vi "Launch Subordinate and Add.vi"(6 "PanelIndex":i32, 7 "Identifier":string, 8 "error in (no error)":errorcluster, 9 "Panel":refnum<class "Panel.lvclass">, 10 "Nested Panel Actor":refnum<class "Panel Actor.lvclass">, 11 "Managed Actor in":refnum<class "Managed Actor.lvclass">) -> (0 "error out":errorcluster, 3 "Managed Actor out":refnum<class "Managed Actor.lvclass">)   [LabVIEW 2023, in "Engine.lvlib" / "Managed Actor.lvlib" / "Managed Actor.lvclass"]
doc: "<b>Launch Subordiate and Add</b>\nThis routine searches for an existing record of the specific subordinate being called. This prevents duplicate references to the same actor being launched.\n\nif no duplicate is found, <b>Launch Subordinate</b> is called, and the returned record is added to the map using <b>Add Subordinate</b>"
uses:
  Library/Managed Actor.lvclass
  builds/Framework/Panel Manager.lvlibp/Panel/Panel/Panel.lvclass
  builds/Framework/Panel Manager.lvlibp/Library/Panel Actor.lvclass
  Engine/Library/Engine.lvclass
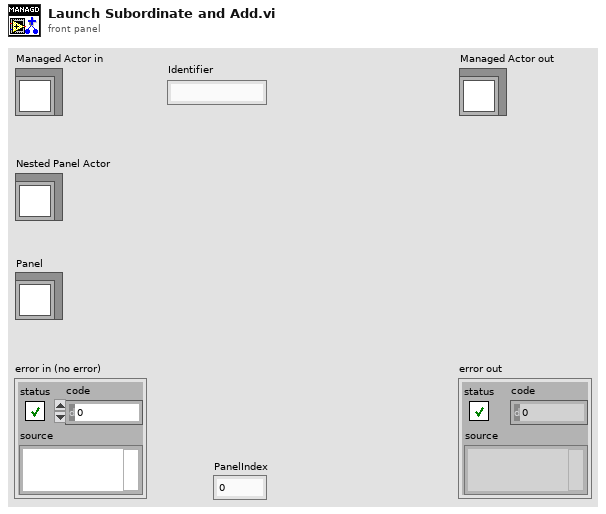
[diagram p1: front panel]
types:
  T1 = typedef "Engine.lvlib/Managed Actor.lvlib/Managed Actor.lvclass/Subordinate.ctl" = cluster{"Identifier":string, "Queue":refnum<class "Message Enqueuer.lvclass">, "PanelIndex":i32}
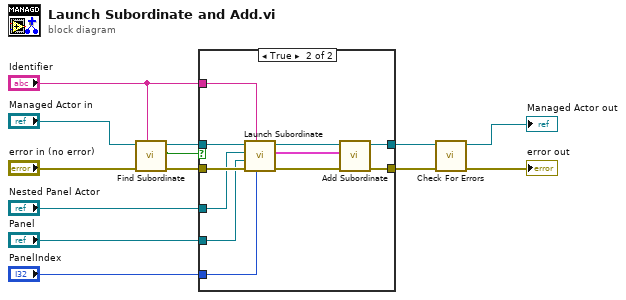
[diagram p0: block diagram]
diagram:
  n1 = call "Find Subordinate.vi"("Identifier"="Identifier", "error in (no error)"="error in (no error)", "Managed Actor in"="Managed Actor in") -> ("error out"=w9:errorcluster, "not found?"=w11:bool, "Managed Actor out"=w10:refnum<class "Managed Actor.lvclass">)  [unwired: 4 in, 2 out]
  n2 = case shown="True" w11 {
    tunnel: w10 -> [w15 w23]
    tunnel: w9 -> [w14 w22]
    tunnel: [w15 w21] -> w2
    tunnel: [w14 w20] -> w8
    tunnel: "Identifier" -> [_ w19]
    tunnel: "PanelIndex" -> [_ w18]
    tunnel: "Nested Panel Actor" -> [_ w17]
    tunnel: "Panel" -> [_ w16]
    frame False {
    }
    frame True {
      n3 = call "Launch Subordinate.vi"("PanelIndex"=w18, "Identifier"=w19, "error in (no error)"=w22, "Panel"=w16, "Nested Panel Actor"=w17, "Managed Actor in"=w23) -> ("error out"=w26:errorcluster, "Subordinate"=w24:T1, "Managed Actor out"=w25:refnum<class "Managed Actor.lvclass">)  [unwired: 3 in]
      n4 = call "Add Subordinate.vi"("error in (no error)"=w26, "Subordinate"=w24, "Managed Actor in"=w25) -> ("error out"=w20:errorcluster, "Managed Actor out"=w21:refnum<class "Managed Actor.lvclass">)  [unwired: 7 in]
    }
  }
  n5 = call "Check For Errors.vi"("error in"=w8, "Engine in"=w2) -> ("error out"=→"error out":errorcluster, "Engine out"=→"Managed Actor out":refnum<class "Managed Actor.lvclass">)  [unwired: 8 in]
